vi "Create Transfer Sections.vi"(7 "GUID (Default Section)":string="03D3BB89-1485-13A6-56005DE6430FF8B7", 8 "error in (no error)":errorcluster, 10 "Transfer Configurations":refnum<class "Transfer Configuration.lvclass">[](array[class]), 11 "Item Ref in":T1 format="%.0x") -> (0 "error out":errorcluster, 2 "Transfer Section refs":T1[](array[typedef]) format="%.0x", 3 "Item Ref out":T1 format="%.0x")   [LabVIEW 2017, in "DSF System Explorer.lvlib"]
uses:
  DSF System Explorer.lvlib
  <vilib>/NI Veristand/Custom Device API/Custom Device Item Ref.ctl
  DSF Core.lvlibp/Classes/Configuration/Base/Transfer/Transfer Configuration.lvclass
  <vilib>/NI Veristand/Custom Device API/Custom Device API.lvlib
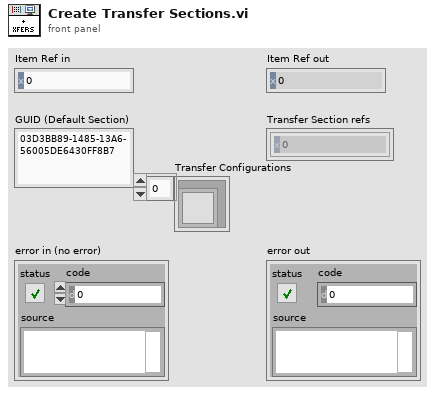
[diagram p1: front panel]
types:
  T1 = typedef "Custom Device API.lvlib/Custom Device Item Ref.ctl" = u64
  T2 = typedef "DSF Core.lvlibp/DSF Core Transfer Configuration.ctl" = cluster{"name":string}
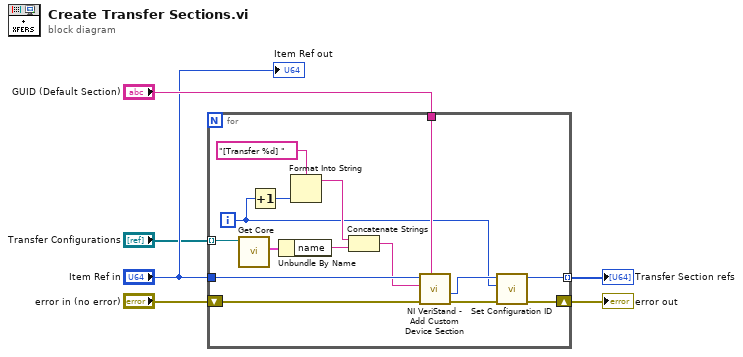
[diagram p0: block diagram]
diagram:
  n1 = for {
    tunnel: "Transfer Configurations" -> [w9] mode=indexing
    tunnel: "Item Ref in" -> [w21]
    shift-right: [w14] -> w6
    shift-left: "error in (no error)" -> [w20]
    tunnel: [w13] -> w5 mode=indexing
    tunnel: "GUID (Default Section)" -> [w12]
    i -> [w10]
    n2 = call "Get Core.vi"("Transfer Configuration in"=w9) -> ("core"=w8:T2)  [unwired: 8 in, 2 out]
    n3 = Increment(x=w10) -> (x+1=w11:i32)
    n4 = Unbundle By Name(w8) -> ("name"=w7:string)
    n5 = Format Into String(format string="[Transfer %d] ", w11) -> (resulting string=w18:string)  [unwired: 2 in, 1 out]
    n6 = Concatenate Strings(w18, w7) -> (w17:string)
    n7 = call <vilib>:"NI VeriStand - Add Custom Device Section.vi"("GUID (Default Section)"=w12, "error in (no error)"=w20, "Section Name"=w17, "Parent Ref in"=w21) -> ("error out"=w19:errorcluster, "Section Ptr"=w15:T1)  [unwired: 4 in, 2 out]
    n8 = call "Set Configuration ID.vi"("error in (no error)"=w19, "Configuration ID"=w10, "Item Ref in"=w15) -> ("error out"=w14:errorcluster, "Item Ref out"=w13:T1)  [unwired: 7 in]
  }
  "error out" <- w6
  "Transfer Section refs" <- w5
  "Item Ref out" <- "Item Ref in"
